vi "Tach Speed from Pulse Position (No State).vi"(6 "state in":T1, 7 "Empty Block Cutoff":i32, 11 "speed position info":T2) -> (3 "RPM":dbl, 4 "state out":T1)   [LabVIEW 2017, in "VibrationAnalysisFunctions.lvlib"]
uses:
  <vilib>/addons/InsightCM/Utilities/Analysis/Vibration/VibrationAnalysisFunctions.lvlib
  <vilib>/addons/Sound and Vibration/Order Analysis/Misc/OAT Position Info.ctl
  <vilib>/Analysis/baseanly.llb/Mean (DBL).vi
  <vilib>/Analysis/NI_AALBase.lvlib
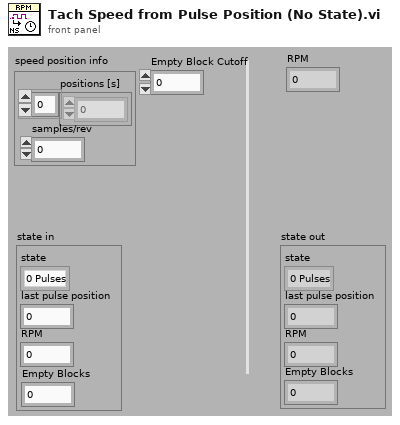
[diagram p1: front panel]
types:
  T1 = cluster{"state":enum16{"0 Pulses", "1 Pulse", "2+ Pulses"}, "last pulse position":dbl, "RPM":dbl, "Empty Blocks":i32}
  T2 = typedef "OAT Position Info.ctl" = cluster{"positions [s]":dbl[], "samples/rev":dbl}
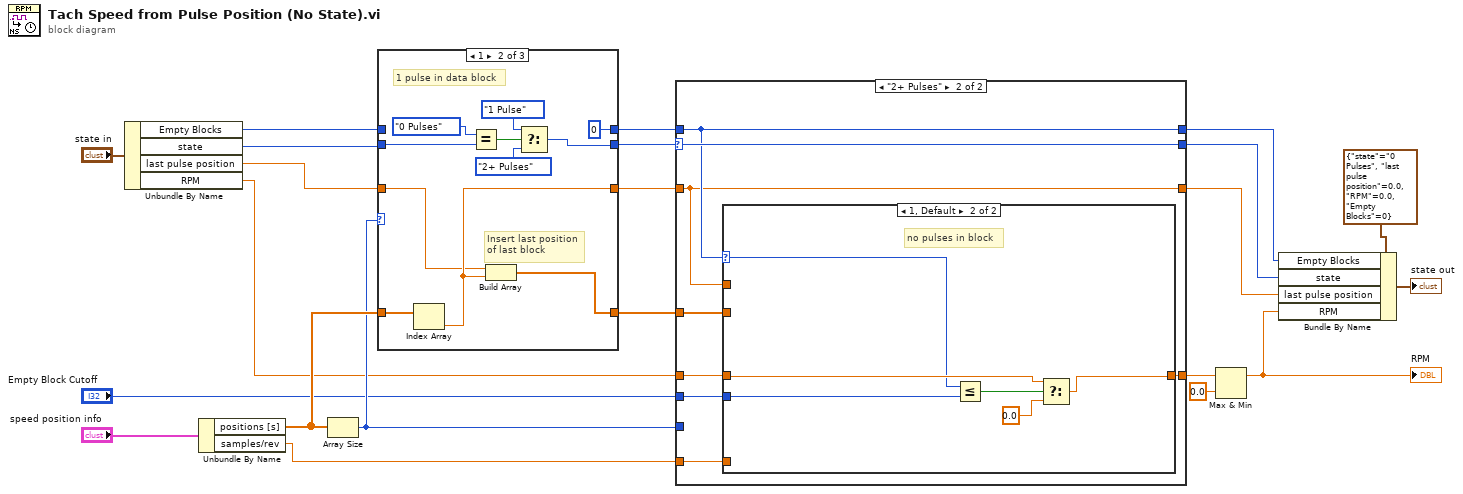
[diagram p0: block diagram]
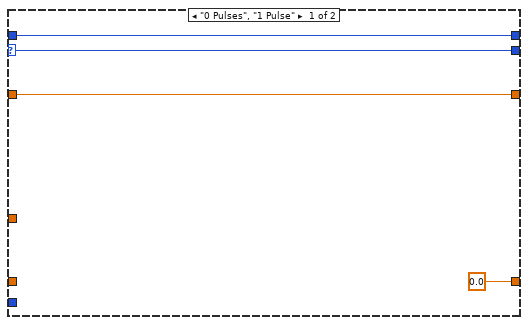
[diagram p2: hidden frame]
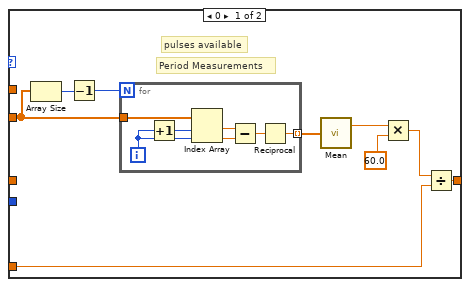
[diagram p3: hidden frame]
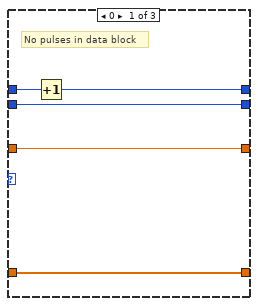
[diagram p4: hidden frame]
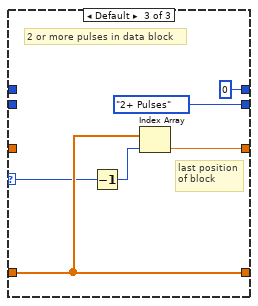
[diagram p5: hidden frame]
diagram:
  n1 = Unbundle By Name("state in") -> ("Empty Blocks"=w8:i32, "state"=w13:enum16{"0 Pulses", "1 Pulse", "2+ Pulses"}, "last pulse position"=w12:dbl, "RPM"=w11:dbl)
  n2 = Unbundle By Name("speed position info") -> ("positions [s]"=w19:dbl[], "samples/rev"=w4:dbl)
  n3 = Array Size(array=w19) -> (size(s)=w17:i32)
  n4 = case shown="1" w17 {
    selector: w17 -> [_ _ w43]
    tunnel: w12 -> [w26 w35 _]
    tunnel: [w26 w36 w41] -> w16
    tunnel: w13 -> [w27 w33 _]
    tunnel: [w27 w29 enum16{"0 Pulses", "1 Pulse", "2+ Pulses"}."2+ Pulses" ("Enum")] -> w15
    tunnel: w19 -> [w25 w38 w44]
    tunnel: [w25 w37 w44] -> w14
    tunnel: w8 -> [w24 _ _]
    tunnel: [w23 0 0] -> w7
    frame 0 {
      # "No pulses in data block"
      n5 = Increment(x=w24) -> (x+1=w23:i32)
    }
    frame 1 {
      # "Insert last position\nof last block"
      # "1 pulse in data block"
      n6 = Index Array(array=w38) -> (element=w36:dbl)  [unwired: 1 in]
      n7 = Equal?(x=enum16{"0 Pulses", "1 Pulse", "2+ Pulses"}."0 Pulses" ("Enum"), y=w33) -> (x = y?=w32:bool)
      n8 = Build Array(w35, w36) -> (w37:dbl[])
      n9 = Select(t=enum16{"0 Pulses", "1 Pulse", "2+ Pulses"}."1 Pulse" ("Enum"), s=w32, f=enum16{"0 Pulses", "1 Pulse", "2+ Pulses"}."2+ Pulses" ("Enum")) -> (s? t:f=w29:enum16{"0 Pulses", "1 Pulse", "2+ Pulses"})
    }
    frame Default {
      # "last position\nof block"
      # "2 or more pulses in data block"
      n10 = Decrement(x=w43) -> (x-1=w42:i32)
      n11 = Index Array(array=w44, index=w42) -> (element=w41:dbl)
    }
  }
  n12 = case shown="\"2+ Pulses\"" w15 {
    selector: w15 -> [w48 w53]
    tunnel: [0.0 w56] -> w3
    tunnel: w14 -> [_ w55]
    tunnel: w11 -> [_ w49]
    tunnel: w4 -> [_ w54]
    tunnel: w17 -> [_ _]
    tunnel: [w48 w53] -> w20
    tunnel: w16 -> [w47 w50]
    tunnel: [w47 w50] -> w21
    tunnel: w7 -> [w46 w52]
    tunnel: [w46 w52] -> w6
    tunnel: "Empty Block Cutoff" -> [_ w51]
    frame "0 Pulses", "1 Pulse" {
    }
    frame "2+ Pulses" {
      n13 = case shown="1, Default" w52 {
        selector: w52 -> [_ w74]
        tunnel: [w65 w76] -> w56
        tunnel: w55 -> [w64 _]
        tunnel: w54 -> [w63 _]
        tunnel: w51 -> [_ w73]
        tunnel: w50 -> [_ _]
        tunnel: w49 -> [_ w75]
        frame 0 {
          # "pulses available"
          # "Period Measurements"
          n14 = Array Size(array=w64) -> (size(s)=w62:i32)
          n15 = Decrement(x=w62) -> (x-1=w57:i32)
          n16 = for {
            N: w57 -> [_]
            tunnel: w64 -> [w72]
            tunnel: [w71] -> w61 mode=indexing
            i -> [w67]
            n17 = Increment(x=w67) -> (x+1=w68:i32)
            n18 = Index Array(array=w72, index #1=w68, index #2=w67) -> (element #1=w66:dbl, element #2=w69:dbl)
            n19 = Subtract(x=w66, y=w69) -> (x-y=w70:dbl)
            n20 = Reciprocal(x=w70) -> (1/x=w71:dbl)
          }
          n21 = call-poly <vilib>:"Mean.vi"("X"=w61) -> ("mean"=w59:dbl)  [unwired: 1 out]
          n22 = Multiply(x=w59, y=60.0) -> (x*y=w58:dbl)
          n23 = Divide(x=w58, y=w63) -> (x/y=w65:dbl)
        }
        frame 1, Default {
          # "no pulses in block"
          n24 = Less Or Equal?(x=w74, y=w73) -> (x <= y?=w78:bool)
          n25 = Select(t=w75, s=w78, f=0.0) -> (s? t:f=w76:dbl)
        }
      }
    }
  }
  n26 = Max & Min(x=w3, y=0.0) -> (max(x,y)=w2:dbl)  [unwired: 1 out]
  "RPM" <- w2
  n27 = Bundle By Name(cluster=T1 {"state"=enum."0 Pulses", "last pulse position"=0.0, "RPM"=0.0, "Empty Blocks"=0} ("state in"), "Empty Blocks"=w6, "state"=w20, "last pulse position"=w21, "RPM"=w2) -> (→"state out":T1)
